vi "ENPH354_LabSCPE.vi"() -> ()   [LabVIEW 2020]
uses:
  <vilib>/Utility/file.llb/Read Delimited Spreadsheet (DBL).vi
panel:
  out "FF":dbl
  in  "Save Data":path
  out "PCE(n)":dbl
  out "I_m [A]":dbl
  out "V_m [V]":dbl
  out "I_sc [A]":dbl
  out "V_oc [V]":dbl
  out "R_s [Ohm]":dbl
  out "R_sh [Ohm]":dbl
  out "Measurement Data":dbl[][](array[numeric])
  out "IV":cluster{"X":dbl[], "Y":dbl[]}[](graph)
  in  "Open Data":path
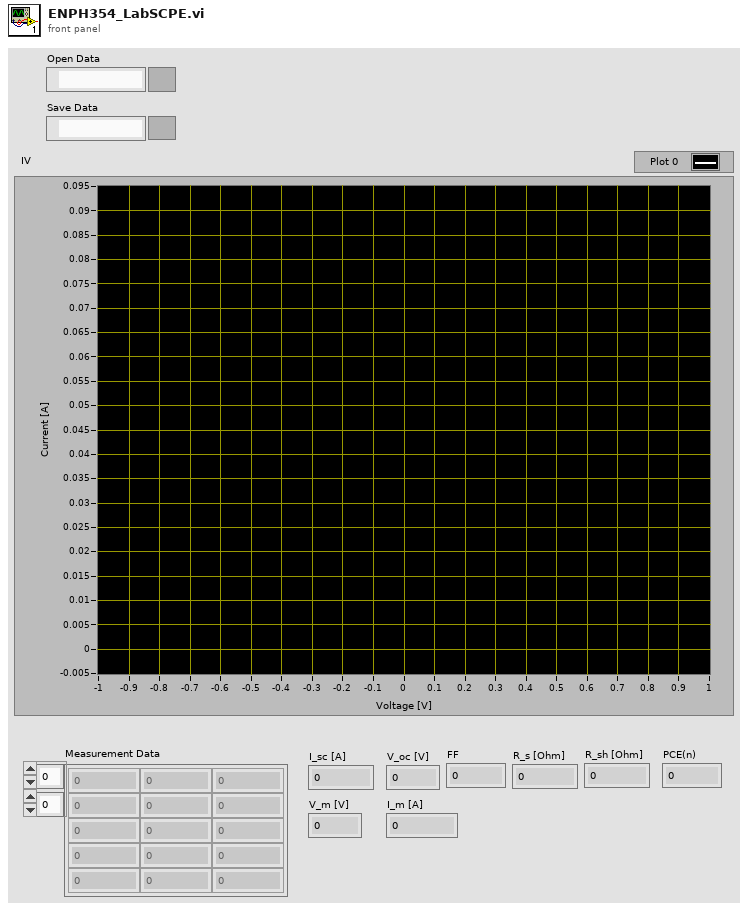
[diagram p1: front panel]
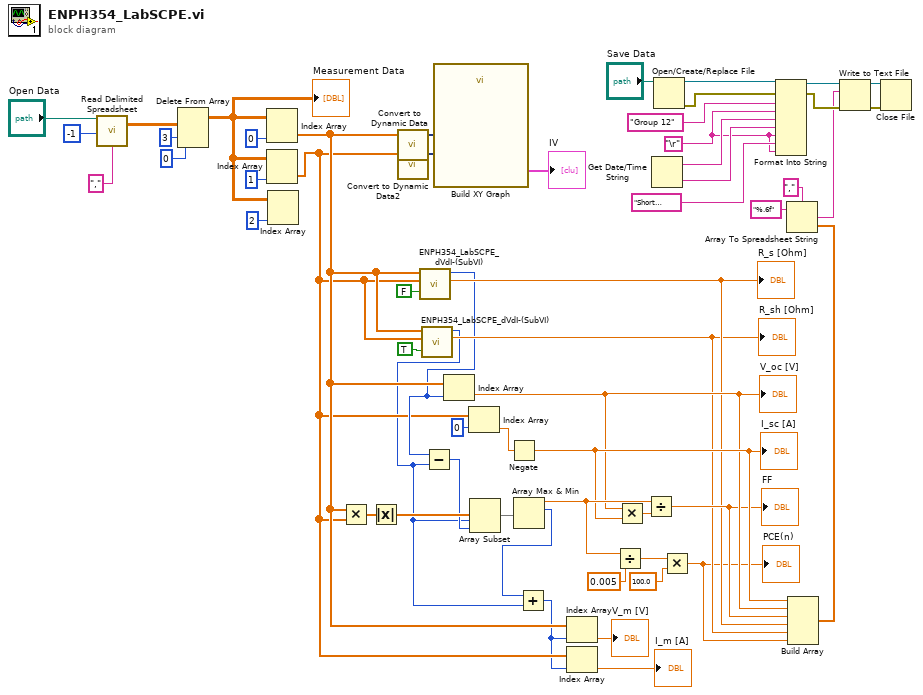
[diagram p0: block diagram]
diagram:
  w29 = "\r"
  n1 = call-poly <vilib>:"Read Delimited Spreadsheet.vi"("file path (dialog if empty)"="Open Data", "number of rows (all:-1)"=-1, "delimiter (\\t)"="," ("delimiter (\\t)")) -> ("all rows"=w53:dbl[][])  [unwired: 7 in, 5 out]
  n2 = Delete From Array(array=w53, length=3, index (row)=0) -> (array with subset deleted=w44:dbl[][])  [unwired: 1 in, 1 out]
  "Measurement Data" <- w44
  n3 = Index Array(array=w44, index (col)=0) -> (element=w22:dbl[])  [unwired: 1 in]
  n4 = Index Array(array=w44, index (col)=1) -> (element=w4:dbl[])  [unwired: 1 in]
  n5 = Index Array(array=w44, index (col)=2 ("disabled index (col)")) -> ()  [unwired: 1 in, 1 out]
  n6 = Multiply(x=w22, y=w4) -> (x*y=w9:dbl[])
  n7 = Absolute Value(x=w9) -> (abs(x)=w8:dbl[])
  n8 = call "Convert to Dynamic Data"("Array"=w22) -> ("Dynamic Data Type"=w46:dynamicdata)  [unwired: 3 in]
  n9 = call "Convert to Dynamic Data2"("Array"=w4) -> ("Dynamic Data Type"=w45:dynamicdata)  [unwired: 3 in]
  n10 = call "ENPH354_LabSCPE_dVdI-(SubVI).vi"("Shunt or Series"=FALSE, "Current in"=w4, "Voltage in"=w22) -> ("dV/dI"=w13:dbl, "IDX"=w7:u8)  [unwired: 7 in]
  "R_s [Ohm]" <- w13
  n11 = call "ENPH354_LabSCPE_dVdI-(SubVI).vi"("Shunt or Series"=TRUE, "Current in"=w4, "Voltage in"=w22) -> ("dV/dI"=w12:dbl, "IDX"=w3:u8)  [unwired: 7 in]
  "R_sh [Ohm]" <- w12
  n12 = Subtract(x=w7, y=w3) -> (x-y=w6:u8)
  n13 = call "Build XY Graph"("Y Input"=w45, "X Input"=w46) -> ("XY Graph"=→"IV":cluster{"X":dbl[], "Y":dbl[]}[])  [unwired: 8 in, 1 out]
  n14 = Index Array(array=w22, index=w7) -> (element=w15:dbl)
  "V_oc [V]" <- w15
  n15 = Index Array(array=w4, index=0) -> (element=w25:dbl)
  n16 = Array Subset(array=w8, index=w3, length=w6) -> (w5:dbl[])
  n17 = Negate(x=w25) -> (-x=w16:dbl)
  "I_sc [A]" <- w16
  n18 = Array Max & Min(array=w5) -> (max value=w17:dbl, max index (indices)=w2:i32)  [unwired: 2 out]
  n19 = Add(x=w2, y=w3) -> (x+y=w1:i32)
  n20 = Index Array(array=w22, index=w1) -> (element=→"V_m [V]":dbl)
  n21 = Index Array(array=w4, index=w1) -> (element=→"I_m [A]":dbl)
  n22 = Divide(x=w17, y=0.005) -> (x/y=w19:dbl)
  n23 = Multiply(x=w15, y=w16) -> (x*y=w23:dbl)
  n24 = Divide(x=w17, y=w23) -> (x/y=w14:dbl)
  "FF" <- w14
  n25 = Get Date/Time String() -> (date string=w35:string, time string=w34:string)  [unwired: 3 in]
  n26 = Open/Create/Replace File(file path (use dialog)="Save Data") -> (refnum out=w43:refnum<file>, error out=w40:errorcluster)  [unwired: 5 in, 1 out]
  n27 = Multiply(x=w19, y=100.0) -> (x*y=w11:dbl)
  "PCE(n)" <- w11
  n28 = Format Into String(initial string=w43, error in=w40, "Group 12" ("input 1"), w29, w35, w34, w29, "Short Circuit Current [A], Open-circuit Voltage [V], Fill Factor, Series Resistance [Ohm], Shunt Resistance [Ohm], Power Conversion Efficiency [%] ", w29) -> (resulting string=w42:refnum<file>, error out=w39:errorcluster)  [unwired: 1 in]
  n29 = Build Array(w16, w15, w14, w13, w12, w11) -> (w10:dbl[])
  n30 = Array To Spreadsheet String(delimiter (Tab)=",", array=w10, 3:"%.6f" ("format string")) -> (spreadsheet string=w32:string)
  n31 = Write to Text File(file (use dialog)=w42, text=w32, error in=w39) -> (refnum out=w41:refnum<file>, error out=w38:errorcluster)  [unwired: 1 in, 1 out]
  n32 = Close File(refnum=w41, error in=w38) -> ()  [unwired: 2 out]
